vi "SiosIfmI2CReadBuffer.vi"(1 "Device Number":i32) -> (0 "i2c Buffer":string)   [LabVIEW 2009]
uses:
  siosifm.dll
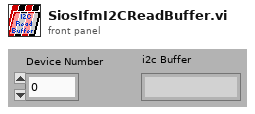
[diagram p1: front panel]
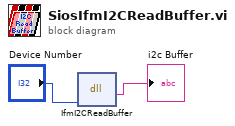
[diagram p0: block diagram]
diagram:
  n1 = dll-call lib="C:/WORK/Artem/RE-10/SIOS_IfmDLL/siosifm.dll" fn="IfmI2CReadBuffer"("devNumber"="Device Number") -> ("i2c Buffer"=→"i2c Buffer":string)  [unwired: 4 in, 2 out]
